vi "globalSetUp.vi"(8 "error in":errorcluster, 11 "testcase-CSMSubModule in":refnum<class "testcase-CSMSubModule.lvclass">) -> (0 "error out":errorcluster, 3 "testcase-CSMSubModule out":refnum<class "testcase-CSMSubModule.lvclass">)   [LabVIEW 2017, in "testcase-CSMSubModule.lvclass"]
uses:
  testcase-CSMSubModule.lvclass
  testcase-CSMSubModule.lvclass/testcase-CSMSubModule.ctl
  <vilib>/addons/_JKI Toolkits/VI Tester/TestCase.llb/TestCase.lvclass
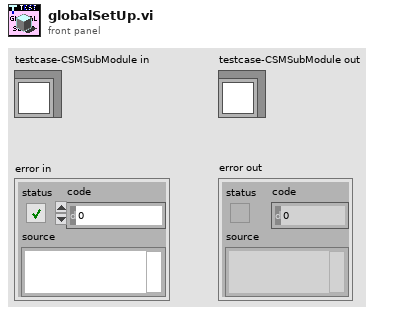
[diagram p1: front panel]
types:
  T1 = cluster{"name":string, "num":i32, "prototype":string[]}[]
  T2 = cluster{"prototype":string, "name":string, "num":i32, "index":i32}[]
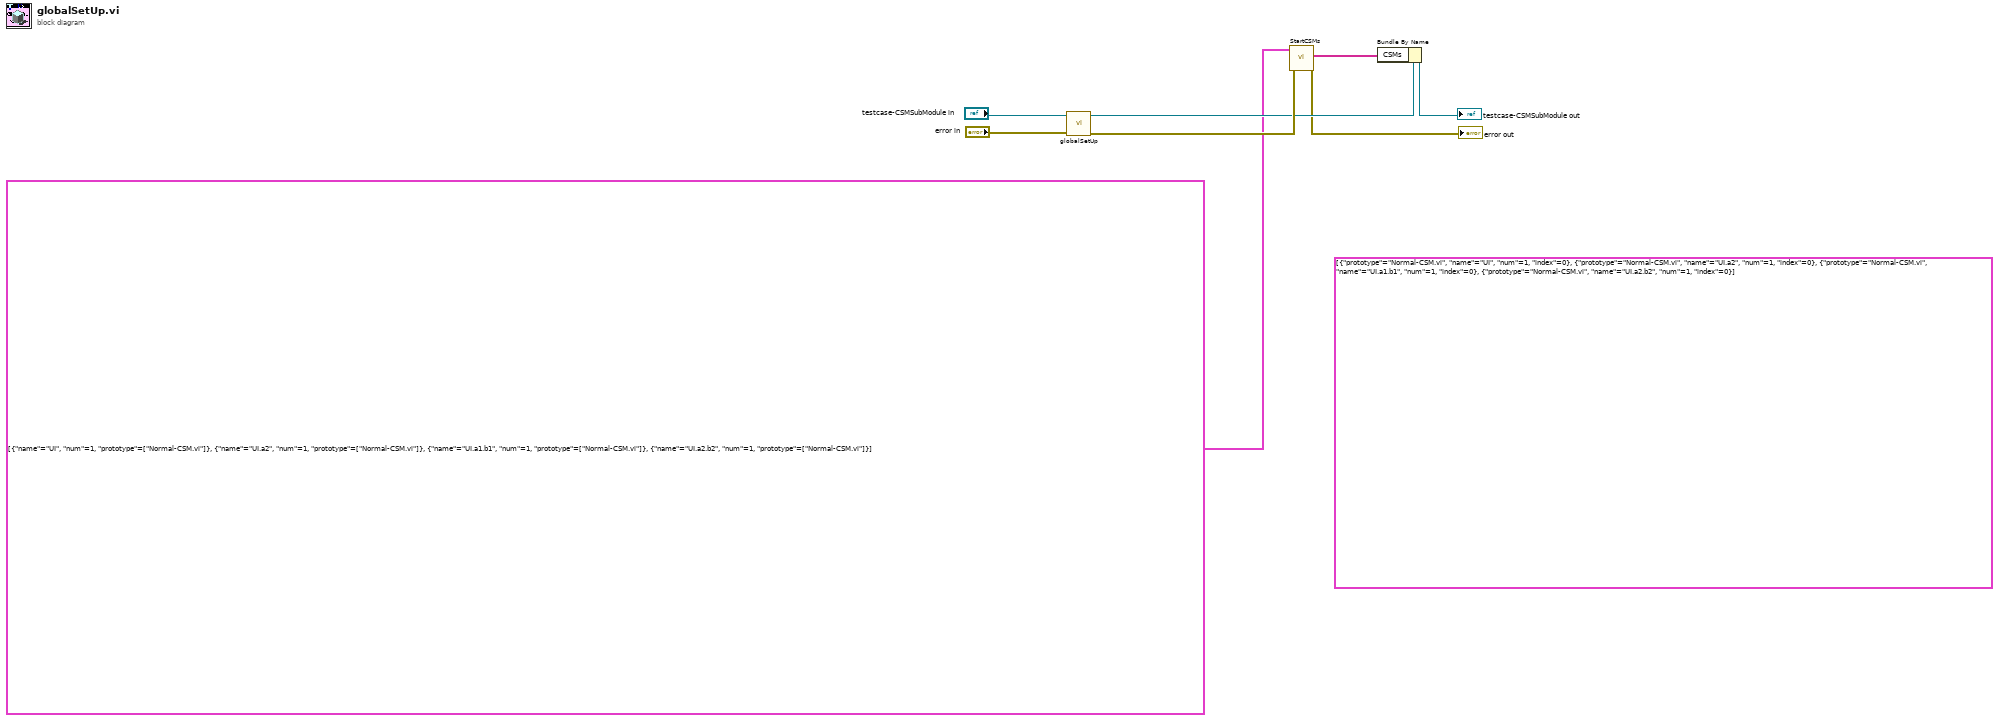
[diagram p0: block diagram]
diagram:
  (unwired) T2 [{"prototype"="Normal-CSM.vi", "name"="UI", "num"=1, "index"=0}, {"prototype"="Normal-CSM.vi", "name"="UI.a2", "num"=1, "index"=0}, {"prototype"="Normal-CSM.vi", "name"="UI.a1.b1", "num"=1, "index"=0}, {"prototype"="Normal-CSM.vi", "name"="UI.a2.b2", "num"=1, "index"=0}]
  n1 = call-parent "globalSetUp.vi"("error in (no error)"="error in", "TestCase in"="testcase-CSMSubModule in") -> ("error out"=w6:errorcluster, "TestCase out"=w5:refnum<class "testcase-CSMSubModule.lvclass">)  [unwired: 8 in]
  n2 = call "StartCSMs.vi"("error in"=w6, "Array"=T1 [{"name"="UI", "num"=1, "prototype"=["Normal-CSM.vi"]}, {"name"="UI.a2", "num"=1, "prototype"=["Normal-CSM.vi"]}, {"name"="UI.a1.b1", "num"=1, "prototype"=["Normal-CSM.vi"]}, {"name"="UI.a2.b2", "num"=1, "prototype"=["Normal-CSM.vi"]}]) -> ("error out"=→"error out":errorcluster, "CSMs"=w2:string[])  [unwired: 8 in]
  n3 = Bundle By Name(cluster=w5, "CSMs"=w2) -> (→"testcase-CSMSubModule out":refnum<class "testcase-CSMSubModule.lvclass">)
